vi "multi-mode-acquisition.vi"() -> ()   [LabVIEW 2014]
uses:
  Globals/Initilize Globals.vi
  <vilib>/vision/Image Controls.llb/IMAQ Image.ctl
  Glimpse-master/Glimpse core/Seq file v 1/Offset.ctl
  Glimpse-master/Glimpse core/Seq file v 1/file number.ctl
  Glimpse-master/Glimpse core/Seq file v 1/Offset table.ctl
  SubVIs/ctt's/Video acquisition state1.ctl
  Shutter Control/Shutter SubVis/Global Shutter Variables - SubVI.vi
  Shutter Control/Shutter SubVis/ctts/user event shutter global.ctl
  TIRF Lock/Globals/autofocus-globals.vi
  Stage Control/stage-controller-globals.vi
  File Directory/File-Locations-Global.vi
  Shutter Control/Shutter SubVis/ctts/laser shutters.ctl
  SubVIs/ctt's/Camera Setup Acquisition.ctl
  SubVIs/ctt's/acquisition protocol.ctl
  SubVIs/ctt's/Image size and binning.ctl
  SubVIs/ctt's/acquisition protocol multimode.ctl
panel:
  in  "Acquisition directory root path":path=path "c:/scratch"
  in  "Max Cycles":i32
  in  "Cycle Interval (s)":dbl format="%_2g"
  in  "Scan Fields":bool
  in  "Scan Field Options":T1(radio)
  in  "Max. number of acquisition files":i8(slide)=10 scale=0.0..50.0
  in  "Acquisition Protocol":T2
  in  "Quit":bool
  in  "Start":bool
  in  "Acquisition Parameters":T5={"Readout Mode"=enum."Image", "Set Acquisition Mode"=enum."Single Scan", "Trigger Mode"=enum."Internal", "Exposure Time (sec)"=1.0, "Accumulation Cycle (s)"=0.0, "Kinetic Cycle Time (s)"=1.0, "Number of Kinetics"=1, "Number of Accumulations"=1, "Set VS Speed"=1.0, "Pixel Rate"=enum."Standard CCD 3 Mhz 14 bits", "V Shift Amplitude"=enum."+1", "Preamp Gain"=enum."1.0", "Single Track Settings"={"centre"=0, "height"=1}, "EM CCD Gain"=300, "High Capacity?"=FALSE} {"EM CCD Gain" scale=0.01..300.0; "Single Track Settings"."centre" min=0 max=1024; "Single Track Settings"."height" min=1 max=1024; "Exposure Time (sec)" scale=0.001..10.0 scale format="%#_1g"}
  in  "Image Size":T6={"H Bin"=1.0, "V Bin"=1.0, "Left"=1.0, "Right"=1024.0, "Top"=1.0, "Bottom"=1024.0} {"V Bin" min=0.0; "H Bin" min=0.0 step=1.0}
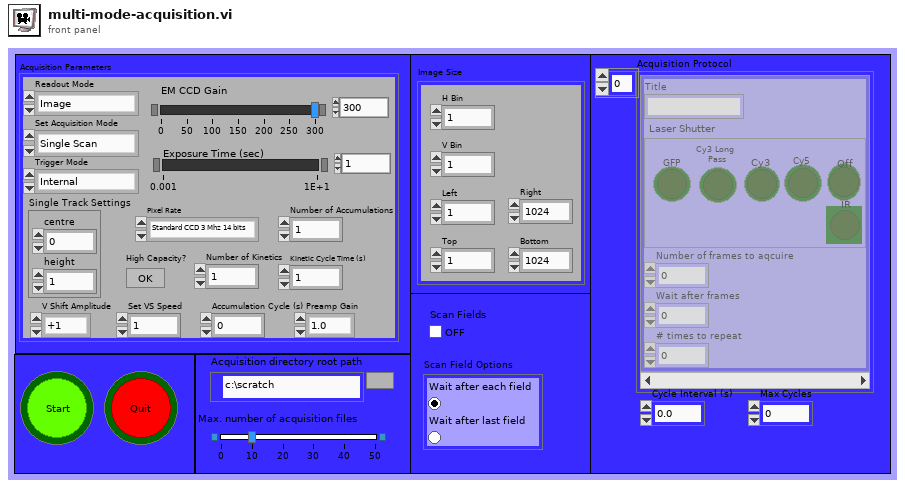
[diagram p1: front panel]
types:
  T1 = enum32{"Wait after each field", "Wait after last field"}
  T2 = typedef "acquisition protocol multimode.ctl" = T3[]
  T3 = typedef "acquisition protocol.ctl" = cluster{"Title":string, "Laser Shutter":T4, "Number of frames to aqcuire":dbl, "Wait after frames":dbl, "# times to repeat":u32}
  T4 = typedef "laser shutters.ctl" = enum32{"No Selection", "GFP", "Cy3 Long \nPass", "Cy3", "Cy5", "Off", "IR"}
  T5 = typedef "Camera Setup Acquisition.ctl" = cluster{"Readout Mode":enum16{"Full Vertical Binning", "Multi-Track", "Random-Track", "Single-Track", "Image"}, "Set Acquisition Mode":enum16{"(do nothing)", "Single Scan", "Accumulate", "Kinetics", "Fast Kinetics", "Run till abort"}, "Trigger Mode":enum16{"Internal", "External"}, "Exposure Time (sec)":sgl, "Accumulation Cycle (s)":dbl, "Kinetic Cycle Time (s)":dbl, "Number of Kinetics":i32, "Number of Accumulations":i32, "Set VS Speed":dbl, "Pixel Rate":enum16{"EM CCD 10 Mhz 14 bits", "EM CCD 5 Mhz 14 bits", "EM CCD 3 Mhz 14 bits", "EM CCD 1 Mhz 16 bits", "Standard CCD 3 Mhz 14 bits", "Standard CCD 1 Mhz 16 bits"}, "V Shift Amplitude":enum16{"normal", "+1", "+2", "+3", "+4"}, "Preamp Gain":enum16{"1.0", "2.4", "5.0"}, "Single Track Settings":cluster{"centre":i32, "height":i32}, "EM CCD Gain":u16, "High Capacity?":bool}
  T6 = typedef "Image size and binning.ctl" = cluster{"H Bin":dbl, "V Bin":dbl, "Left":dbl, "Right":dbl, "Top":dbl, "Bottom":dbl}
  T7 = enum32{"No Selection", "GFP", "Cy3 Long \nPass", "Cy3", "Cy5", "Off", "IR"}
  T8 = typedef "user event shutter global.ctl" = cluster{"Camera Shutter":bool, "Laser Shutter":enum32{"No Selection", "GFP", "Cy3 Long \nPass", "Cy3", "Cy5", "Off", "IR"}}
  T9 = enum32{"None", "Manual", "Auto - Image analysis", "Auto - Retro-reflection"}
  T10 = cluster{"H Bin":dbl, "V Bin":dbl, "Left":dbl, "Right":dbl, "Top":dbl, "Bottom":dbl}
  T11 = cluster{"Frame Size (bytes)":i32, "Max Time (min)":i32, "Max Frames":i32, "Frames per acquisition file":i32, "Max time (s)":i32, "Max Space Req'd. (Gb)":dbl}
  T12 = typedef "acquisition control.ctl" = cluster{"H Bin":dbl, "V Bin":dbl, "Left":dbl, "Right":dbl, "Top":dbl, "Bottom":dbl}
  T13 = typedef "Video acquisition state1.ctl" = cluster{"Pixel depth":enum32{"8 bits", "16 bits", "Float", "Complex", "RGB Chunky", "Compressed"}, "Width":dbl, "Height":dbl, "Buffer":T14, "Frames Acquired":u32, "Time of 1st frame":dbl, "TTB element zero":u32, "File Offsets Array":T15, "TTB Array":u32[], "Sum Image (for averaging)":T14, "Time at end of last acquisition (ms)":u32, "Flow rate array":dbl[], "Temperature array":dbl[], "Field array":u16[], "Stage xyz array":dbl[][], "Current Filter Wheel Array":string[], "Laser Shutter Array":enum32{"No Selection", "GFP", "Cy3 Long \nPass", "Cy3", "Cy5", "Off", "IR"}[]}
  T14 = typedef "IMAQ Image.ctl" = refnum<image>
  T15 = typedef "Offset table.ctl" = cluster{"offset":T16, "file number":T17}[]
  T16 = typedef "Offset.ctl" = i32
  T17 = typedef "file number.ctl" = u8
  T18 = cluster{"Sequence files directory path":path, "Sequence files refnum array":refnum<file>[]}
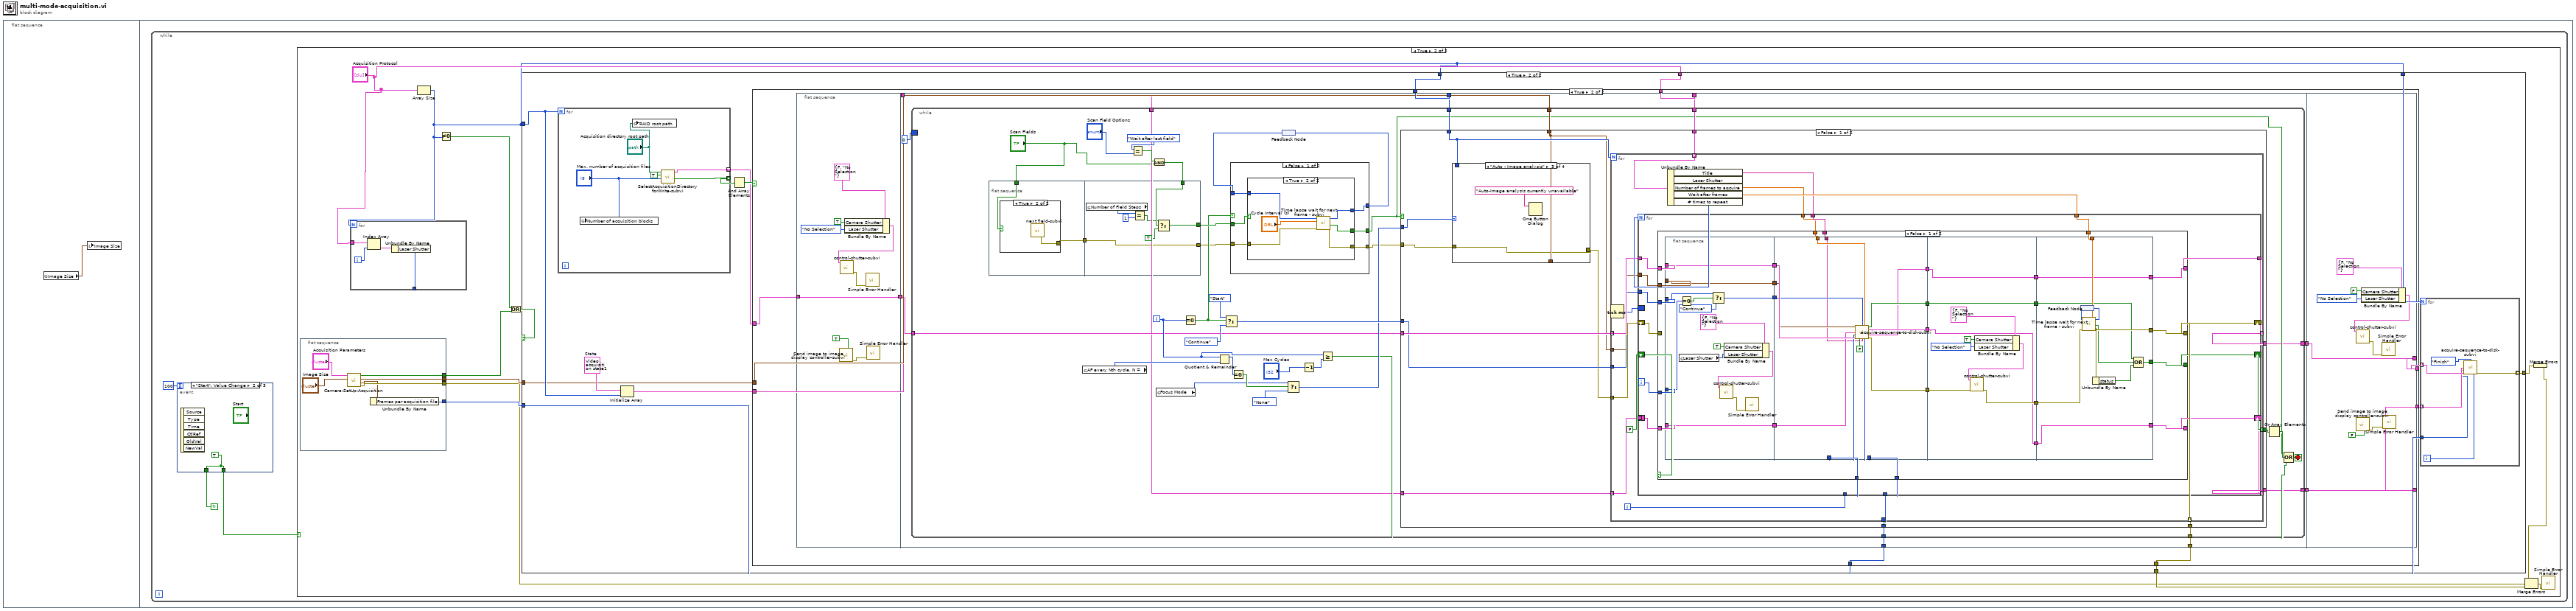
[diagram p0: block diagram]
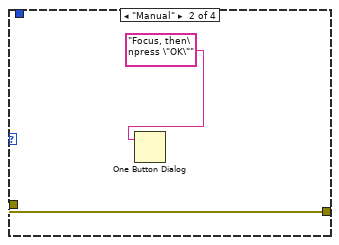
[diagram p7: hidden frame]
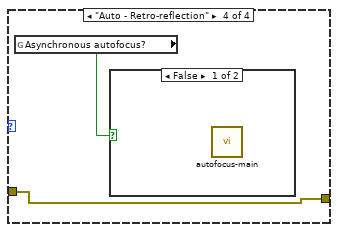
[diagram p8: hidden frame]
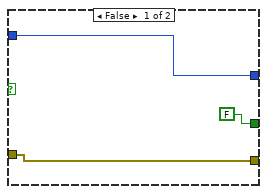
[diagram p11: hidden frame]
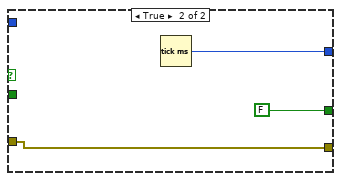
[diagram p12: hidden frame]
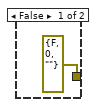
[diagram p13: hidden frame]
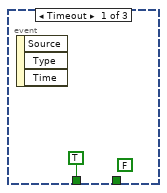
[diagram p14: hidden frame]
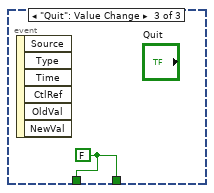
[diagram p15: hidden frame]
diagram:
  n1 = flat-sequence {
    frame #0 {
      n2 = global read "Initilize Globals.vi" "Image Size"() -> (w1:T10)
      n3 = local write "Image Size"(w1) -> ()
    }
    frame #1 {
      n4 = while {
        stop <- w3 continue-if-true
        n5 = event shown="[1] \"Start\": Value Change" {
          selector: _ -> [_ _ _]
          dyn-events: _ -> [_ _ _]
          timeout: 100 -> [_ _ _]
          tunnel: [TRUE w296 w297] -> w3
          tunnel: [_ w296 w297] -> w2
          event Timeout {
            (unwired) FALSE
            n6 = event-data() -> ()  [unwired: 1 in, 3 out]
          }
          event "Start": Value Change {
            w296 = TRUE
            n7 = event-data() -> ()  [unwired: 1 in, 6 out]
          }
          event "Quit": Value Change {
            w297 = FALSE
            n8 = event-data() -> ()  [unwired: 1 in, 6 out]
          }
        }
        n9 = case shown="True" w2 {
          frame False {
          }
          frame True {
            n10 = flat-sequence {
              tunnel: [w292] -> w15
              tunnel: [w291] -> w9
              tunnel: [w289] -> w13
              tunnel: [w288] -> w10
              frame #0 {
                n11 = call "Camera-SetUp-Acquisition.vi"("Image Size"="Image Size", "Acquisition Parameters"="Acquisition Parameters") -> ("Error Out"=w291:errorcluster, "File properties"=w290:T11, "Image Size Out"=w289:T12, "Continue with acq?"=w292:bool)  [unwired: 6 in]
                n12 = Unbundle By Name(w290) -> ("Frames per acquisition file"=w288:i32)
              }
            }
            n13 = Array Size(array="Acquisition Protocol") -> (size(s)=w7:i32)
            n14 = for {
              N: w7 -> [_]
              tunnel: "Acquisition Protocol" -> [w20]
              tunnel: [w17] -> _
              i -> [w19]
              n15 = Index Array(array=w20, index=w19) -> (element=w18:T3)
              n16 = Unbundle By Name(w18) -> ("Laser Shutter"=w17:T4)
            }
            n17 = Not Equal To 0?(x=w7) -> (x != 0?=w14:bool)
            n18 = Or(x=w14, y=w15) -> (x .or. y?=w16:bool)
            n19 = case shown="True" w16 {
              tunnel: w7 -> [_ w35]
              tunnel: w13 -> [_ w31]
              tunnel: "Acquisition Protocol" -> [_ w30]
              tunnel: w7 -> [_ w29]
              tunnel: [_ w28] -> w12
              tunnel: w7 -> [_ w27]
              tunnel: w10 -> [_ w21]
              tunnel: [_ w24] -> w5
              frame False {
              }
              frame True {
                w34 = T13 {"Pixel depth"=enum."8 bits", "Width"=0.0, "Height"=0.0, "Buffer"=refnum, "Frames Acquired"=0, "Time of 1st frame"=0.0, "TTB element zero"=0, "File Offsets Array"=[], "TTB Array"=[], "Sum Image (for averaging)"=refnum, "Time at end of last acquisition (ms)"=0, "Flow rate array"=[], "Temperature array"=[], "Field array"=[], "Stage xyz array"=[], "Current Filter Wheel Array"=[], "Laser Shutter Array"=[]}  # State
                n20 = for {
                  N: w35 -> [_]
                  tunnel: [w285] -> w33 mode=indexing
                  tunnel: [w284] -> w26 mode=indexing
                  n21 = global write "Initilize Globals.vi" "Number of acquisition blocks"("Max. number of acquisition files") -> ()
                  n22 = global write "File-Locations-Global.vi" "RAID root path"("Acquisition directory root path") -> ()
                  n23 = call "SelectAcquisitionDirectoryforWrite-subvi.vi"("Number of acquisition files"="Max. number of acquisition files", "Autostart?"=TRUE, "Acquisition directory root path"="Acquisition directory root path") -> ("OK?"=w285:bool, "Sequence files handle"=w284:T18)  [unwired: 7 in]
                }
                n24 = Initialize Array(w34, w35) -> (w25:T13[])
                n25 = And Array Elements(Boolean array=w33) -> (logical AND=w32:bool)
                n26 = case shown="True" w32 {
                  tunnel: w31 -> [_ w55]
                  tunnel: w30 -> [_ w54]
                  tunnel: w29 -> [_ w53]
                  tunnel: [_ w52] -> w28
                  tunnel: w26 -> [w43 w50]
                  tunnel: w25 -> [w42 w49]
                  tunnel: w21 -> [_ w48]
                  tunnel: [w42 w46] -> w23
                  tunnel: [w43 w44] -> w22
                  frame False {
                  }
                  frame True {
                    n27 = flat-sequence {
                      tunnel: [w56] -> w51
                      tunnel: w50 -> [w56]
                      tunnel: w55 -> [w72]
                      tunnel: w54 -> [w71]
                      tunnel: w53 -> [w70]
                      tunnel: [w69] -> w52
                      tunnel: w51 -> [w68]
                      tunnel: w49 -> [w67]
                      tunnel: w48 -> [w66]
                      tunnel: [w65] -> w47
                      tunnel: [w64] -> w45
                      tunnel: w47 -> [w275]
                      tunnel: [w275] -> w46
                      tunnel: w45 -> [w274]
                      tunnel: [w274] -> w44
                      frame #0 {
                        n28 = call "Send image to image display controller-subvi.vi"("Start display controller?"=TRUE) -> ("error out"=w59:errorcluster)  [unwired: 8 in, 1 out]
                        n29 = Bundle By Name(cluster=T8 {"Camera Shutter"=FALSE, "Laser Shutter"=enum."No Selection"} ("Shutter Control"), "Camera Shutter"=TRUE, "Laser Shutter"=T7."No Selection") -> (w61:T8)
                        n30 = call "control-shutter-subvi.vi"("Shutter Control"=w61) -> ("Error Out"=w60:errorcluster)  [unwired: 10 in]
                        n31 = call <vilib>:"Simple Error Handler.vi"("error in (no error)"=w60) -> ()  [unwired: 1 in, 8 out]
                        n32 = call <vilib>:"Simple Error Handler.vi"("error in (no error)"=w59) -> ()  [unwired: 1 in, 8 out]
                      }
                      frame #1 {
                        n33 = while {
                          border: 0 -> [_]
                          tunnel: w72 -> [w93]
                          tunnel: w71 -> [w89]
                          tunnel: w70 -> [w88]
                          tunnel: [w85] -> w69
                          tunnel: w68 -> [w83]
                          tunnel: w67 -> [w80]
                          tunnel: w66 -> [w79]
                          tunnel: [w78] -> w65
                          tunnel: [w77] -> w64
                          i -> [w92]
                          stop <- w86 stop-if-true
                          n34 = flat-sequence {
                            tunnel: "Scan Fields" -> [w264]
                            tunnel: [w263] -> w107
                            tunnel: w108 -> [w272]
                            tunnel: w107 -> [w271]
                            tunnel: [w271] -> w91
                            tunnel: [w270] -> w106
                            frame #0 {
                              n35 = case shown="True" w264 {
                                tunnel: [errorcluster {"status"=FALSE, "code"=0, "source"=""} ("Error Out") w266] -> w263
                                frame False {
                                }
                                frame True {
                                n36 = call "next field-subvi.vi"() -> ("Error Out"=w266:errorcluster)  [unwired: 11 in]
                                }
                              }
                            }
                            frame #1 {
                              n37 = global read "stage-controller-globals.vi" "Number of Field Steps"() -> (w268:u32)
                              n38 = Equal?(x=w268, y=u32 1) -> (x = y?=w269:bool)
                              n39 = Select(t=w269, s=w272, f=TRUE) -> (s? t:f=w270:bool)
                            }
                          }
                          n40 = global read "autofocus-globals.vi" "AF every Nth cycle, N ="() -> (w100:u8)
                          n41 = Equal?(x=T1."Wait after last field" ("y"), y="Scan Field Options") -> (x = y?=w111:bool)
                          n42 = And(x=w111, y="Scan Fields") -> (x .and. y?=w108:bool)
                          n43 = global read "autofocus-globals.vi" "Focus Mode"() -> (w98:T9)
                          n44 = Equal To 0?(x=w92) -> (x = 0?=w103:bool)
                          n45 = Quotient & Remainder(x=w92, y=w100) -> (x-y*floor(x/y)=w102:i32)  [unwired: 1 out]
                          n46 = Select(t=enum16{"Start", "Continue", "Finish"}."Start" ("Operation"), s=w103, f=enum16{"Start", "Continue", "Finish"}."Continue" ("Operation")) -> (s? t:f=w97:enum16{"Start", "Continue", "Finish"})
                          n47 = Equal To 0?(x=w102) -> (x = 0?=w101:bool)
                          n48 = feedback #1() -> (w104:u32)
                          n49 = case shown="False" w103 {
                            tunnel: w106 -> [w250 _]
                            tunnel: [w248 w262] -> w105
                            tunnel: w104 -> [w247 _]
                            tunnel: [w249 FALSE] -> w81
                            tunnel: w91 -> [w246 w260]
                            tunnel: [w245 w260] -> w90
                            frame False {
                              n50 = case shown="True" w250 {
                                tunnel: [FALSE w256] -> w249
                                tunnel: [w252 w258] -> w248
                                tunnel: w247 -> [w252 w259]
                                tunnel: w246 -> [w251 w255]
                                tunnel: [w251 w254] -> w245
                                frame False {
                                }
                                frame True {
                                n51 = call "Time lapse wait for next frame - subvi.vi"("Error In"=w255, "Frame Interval (s)"="Cycle Interval (s)", "Time of last frame in"=w259) -> ("Error Out"=w254:errorcluster, "Stopped?"=w256:bool, "Time of this frame out (ms)"=w258:i32)  [unwired: 5 in, 1 out]
                                }
                              }
                            }
                            frame True {
                              n52 = Tick Count (ms)() -> (millisecond timer value=w262:u32)
                            }
                          }
                          n53 = feedback-in #1(w105) -> ()
                          n54 = Select(t=w98, s=w101, f=T9."None") -> (s? t:f=w96:T9)
                          n55 = Decrement(x="Max Cycles") -> (x-1=w74:i32)
                          n56 = Greater Or Equal?(x=w92, y=w74) -> (x >= y?=w82:bool)
                          n57 = case shown="False" w81 {
                            tunnel: w97 -> [w118 _]
                            tunnel: w96 -> [w125 _]
                            tunnel: w93 -> [w117 _]
                            tunnel: w90 -> [w124 _]
                            tunnel: w89 -> [w123 _]
                            tunnel: w88 -> [w122 _]
                            tunnel: [w121 _] -> w85
                            tunnel: [w120 _] -> w84
                            tunnel: w83 -> [w119 w244]
                            tunnel: w80 -> [w116 w243]
                            tunnel: w79 -> [w115 _]
                            tunnel: [w113 w243] -> w78
                            tunnel: [w112 w244] -> w77
                            frame False {
                              n58 = case shown="\"Auto - Image analysis\"" w125 {
                                tunnel: w117 -> [_ _ _ _]
                                tunnel: w124 -> [w236 w237 w240 w241]
                                tunnel: [w236 w237 w240 w241] -> w114
                                tunnel: w122 -> [_ _ _ _]
                                frame "None", Default {
                                }
                                frame "Manual" {
                                n59 = One Button Dialog(message="Focus, then\npress \"OK\"") -> ()  [unwired: 2 out]
                                }
                                frame "Auto - Image analysis" {
                                n60 = One Button Dialog(message="Auto-Image analysis currently unavailable") -> ()  [unwired: 2 out]
                                }
                                frame "Auto - Retro-reflection" {
                                n61 = global read "autofocus-globals.vi" "Asynchronous autofocus?"() -> (w242:bool)
                                n62 = case shown="False" w242 {
                                frame False {
                                n63 = call "autofocus-main.vi"() -> ()  [unwired: 12 in]
                                }
                                frame True {
                                }
                                }
                                }
                              }
                              n64 = for {
                                N: w122 -> [_]
                                tunnel: w123 -> [w143] mode=indexing
                                tunnel: [w141] -> w121 mode=indexing
                                tunnel: [w140] -> w120 mode=indexing
                                tunnel: w119 -> [w137] mode=indexing
                                tunnel: w118 -> [w134]
                                tunnel: w117 -> [w133]
                                tunnel: w116 -> [w131] mode=indexing
                                tunnel: w115 -> [w130]
                                tunnel: w114 -> [w129]
                                tunnel: [w128] -> w113 mode=indexing
                                tunnel: [w127] -> w112 mode=indexing
                                i -> [w132]
                                n65 = Tick Count (ms)() -> (millisecond timer value=w126:u32)
                                n66 = Unbundle By Name(w143) -> ("Title"=w136:string, "Number of frames to aqcuire"=w135:dbl, "Wait after frames"=w138:dbl, "# times to repeat"=w142:u32)  [unwired: 1 out]
                                n67 = for {
                                N: w142 -> [_]
                                shift-right: [w159] -> w141
                                shift-left: w129 -> [w146]
                                shift-right: [w158] -> w140
                                shift-left: FALSE -> [w157]
                                tunnel: w138 -> [w156]
                                tunnel: w137 -> [w155]
                                tunnel: w136 -> [w154]
                                tunnel: w135 -> [w153]
                                tunnel: w134 -> [w152]
                                tunnel: w133 -> [w151]
                                tunnel: w132 -> [w149]
                                tunnel: w131 -> [w148]
                                tunnel: w130 -> [w147]
                                tunnel: [w144] -> w127
                                border: w126 -> [_]
                                shift-right: [w145] -> w128
                                shift-left: _ -> [_]
                                i -> [w150]
                                n68 = case shown="False" w157 {
                                selector: w157 -> [_ w234]
                                tunnel: [w185 w235] -> w159
                                tunnel: [w184 w234] -> w158
                                tunnel: w156 -> [w182 _]
                                tunnel: w155 -> [w181 w232]
                                tunnel: w154 -> [w179 _]
                                tunnel: w153 -> [w178 _]
                                tunnel: w152 -> [w177 _]
                                tunnel: w151 -> [w176 _]
                                tunnel: w150 -> [w174 _]
                                tunnel: w149 -> [w172 _]
                                tunnel: w148 -> [w170 w233]
                                tunnel: w147 -> [w169 _]
                                tunnel: w146 -> [_ w235]
                                tunnel: [w163 w233] -> w145
                                tunnel: [w160 w232] -> w144
                                frame False {
                                n69 = flat-sequence {
                                tunnel: w181 -> [w193]
                                tunnel: [w193] -> w180
                                tunnel: w177 -> [w191]
                                tunnel: w176 -> [w192]
                                tunnel: [w192] -> w175
                                tunnel: w174 -> [w189]
                                tunnel: [w187] -> w173
                                tunnel: [w186] -> w171
                                tunnel: w170 -> [w186]
                                tunnel: w180 -> [w211]
                                tunnel: w179 -> [w199]
                                tunnel: w178 -> [w202]
                                tunnel: w175 -> [w210]
                                tunnel: w173 -> [w209]
                                tunnel: w172 -> [w207]
                                tunnel: w171 -> [w208]
                                tunnel: w169 -> [w206]
                                tunnel: [w204] -> w168
                                tunnel: [w203] -> w167
                                tunnel: [w201] -> w165
                                tunnel: [w200] -> w162
                                tunnel: [w216] -> w183
                                tunnel: w168 -> [w215]
                                tunnel: w167 -> [w213]
                                tunnel: [w214] -> w166
                                tunnel: w165 -> [w214]
                                tunnel: [w213] -> w164
                                tunnel: w162 -> [w212]
                                tunnel: [w212] -> w161
                                tunnel: [w229] -> w185
                                tunnel: [w227] -> w184
                                tunnel: w183 -> [w226]
                                tunnel: w182 -> [w225]
                                tunnel: w166 -> [w223]
                                tunnel: w164 -> [w222]
                                tunnel: [w222] -> w163
                                tunnel: [w221] -> w160
                                tunnel: w161 -> [w221]
                                frame #0 {
                                n70 = global read "Global Shutter Variables - SubVI.vi" "Laser Shutter"() -> (w196:T7)
                                n71 = Equal To 0?(x=w189) -> (x = 0?=w190:bool)
                                n72 = Select(t=w191, s=w190, f=enum16{"Start", "Continue", "Finish"}."Continue" ("Operation")) -> (s? t:f=w187:enum16{"Start", "Continue", "Finish"})
                                n73 = Bundle By Name(cluster=T8 {"Camera Shutter"=FALSE, "Laser Shutter"=enum."No Selection"} ("Shutter Control"), "Camera Shutter"=TRUE, "Laser Shutter"=w196) -> (w195:T8)
                                n74 = call "control-shutter-subvi.vi"("Shutter Control"=w195) -> ("Error Out"=w194:errorcluster)  [unwired: 10 in]
                                n75 = call <vilib>:"Simple Error Handler.vi"("error in (no error)"=w194) -> ()  [unwired: 1 in, 8 out]
                                }
                                frame #1 {
                                n76 = call "acquire-sequence-to-disk-subvi.vi"("Image Size"=w210, "Operation"=w209, "Number of frames to acquire"=w202, "State In"=w208, "Frames per acquisition file"=w206, "Sequence files handle"=w211, "Pressing stop \nautomatically runs finish?"=FALSE ("Pressing stop automatically runs finish?"), "Display Window Title"=w199, "Display Window Number"=w207) -> ("Done?"=w201:bool, "State Out"=w203:T13, "Sequence files handle out"=w200:T18, "Error Out"=w204:errorcluster)  [unwired: 3 in]
                                }
                                frame #2 {
                                n77 = Bundle By Name(cluster=T8 {"Camera Shutter"=FALSE, "Laser Shutter"=enum."No Selection"} ("Shutter Control"), "Camera Shutter"=TRUE, "Laser Shutter"=T7."No Selection") -> (w218:T8)
                                n78 = call "control-shutter-subvi.vi"("Error In"=w215, "Shutter Control"=w218) -> ("Error Out"=w216:errorcluster)  [unwired: 9 in]
                                }
                                frame #3 {
                                n79 = feedback #2() -> (w230:u32)
                                n80 = call "Time lapse wait for next frame - subvi.vi"("Error In"=w226, "Frame Interval (s)"=w225, "Time of last frame in"=w230) -> ("Error Out"=w229:errorcluster, "Stopped?"=w224:bool, "Time of this frame out (ms)"=w231:i32)  [unwired: 5 in, 1 out]
                                n81 = feedback-in #2(w231) -> ()
                                n82 = Unbundle By Name(w229) -> ("status"=w228:bool)
                                n83 = Compound Arithmetic op=OR(w223, w224, w228) -> (w227:bool)
                                }
                                }
                                }
                                frame True {
                                }
                                }
                                }
                              }
                            }
                            frame True {
                            }
                          }
                          n84 = Or Array Elements(Boolean array=w84) -> (logical OR=w87:bool)
                          n85 = Compound Arithmetic op=OR(w81, w87, w82) -> (w86:bool)
                        }
                      }
                      frame #2 {
                        n86 = call "Send image to image display controller-subvi.vi"("Quit display controller?"=FALSE) -> ("error out"=w278:errorcluster)  [unwired: 8 in, 1 out]
                        n87 = Bundle By Name(cluster=T8 {"Camera Shutter"=FALSE, "Laser Shutter"=enum."No Selection"} ("Shutter Control"), "Camera Shutter"=FALSE, "Laser Shutter"=T7."No Selection") -> (w280:T8)
                        n88 = call "control-shutter-subvi.vi"("Shutter Control"=w280) -> ("Error Out"=w279:errorcluster)  [unwired: 10 in]
                        n89 = call <vilib>:"Simple Error Handler.vi"("error in (no error)"=w279) -> ()  [unwired: 1 in, 8 out]
                        n90 = call <vilib>:"Simple Error Handler.vi"("error in (no error)"=w278) -> ()  [unwired: 1 in, 8 out]
                      }
                    }
                  }
                }
                n91 = for {
                  N: w27 -> [_]
                  tunnel: [w41] -> w24 mode=indexing
                  tunnel: w23 -> [w39] mode=indexing
                  tunnel: w22 -> [w40] mode=indexing
                  tunnel: w21 -> [w36]
                  i -> [w38]
                  n92 = call "acquire-sequence-to-disk-subvi.vi"("Operation"=enum16{"Start", "Continue", "Finish"}."Finish", "State In"=w39, "Frames per acquisition file"=w36, "Sequence files handle"=w40, "Display Window Number"=w38) -> ("Error Out"=w41:errorcluster)  [unwired: 7 in, 3 out]
                }
              }
            }
            n93 = Merge Errors(w5) -> (w6:errorcluster)
            n94 = Merge Errors(w6, w9, w12) -> (w11:errorcluster)
            n95 = call <vilib>:"Simple Error Handler.vi"("error in (no error)"=w11) -> ()  [unwired: 4 in, 5 out]
          }
        }
      }
    }
  }
